vi "Scale Channel (Array).vi"(9 "Data":dbl[](array[numeric]), 10 "Scaling Params":dbl[](array[numeric]), 11 "Scaling Type":T1) -> (1 "Scaled Data":dbl[](array[numeric]))   [LabVIEW 2020, in "VolatusData.lvlib" / "Scaling.lvclass"]
uses:
  Scaling.lvclass
  Scaling.lvclass/Scaling.ctl
  VolatusConfig/Scale Type.ctl
  VolatusConfig/VolatusConfig.lvlib
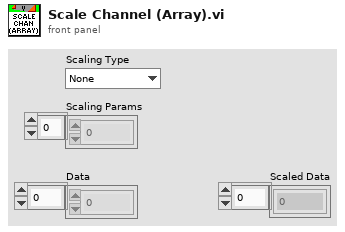
[diagram p1: front panel]
types:
  T1 = typedef "VolatusConfig.lvlib/Scale Type.ctl" = enum16{"None", "Sensor", "Polynomial", "Threshold", "Invert Bool"}
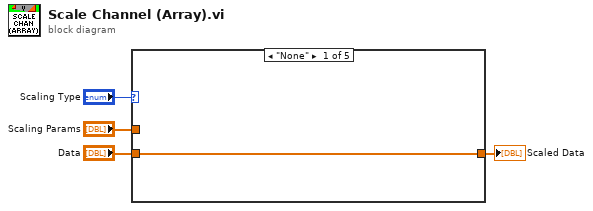
[diagram p0: block diagram]
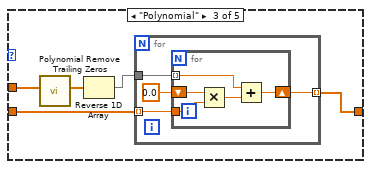
[diagram p3: hidden frame]
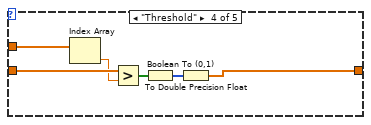
[diagram p4: hidden frame]
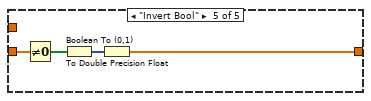
[diagram p5: hidden frame]
diagram:
  n1 = case shown="\"None\"" "Scaling Type" {
    tunnel: "Scaling Params" -> [_ _ w10 w26 _]
    tunnel: "Data" -> [w5 w6 w9 w25 w30]
    tunnel: [w5 w6 w7 w21 w27] -> w1
    frame "None" {
    }
    frame "Sensor" {
      # "#ERROR?\nSensor should be converted to another type."
    }
    frame "Polynomial" {
      n2 = call "Polynomial Remove Trailing Zeros.vi"("Coefficients"=w10) -> ("Used Coefficients"=w11:dbl[])  [unwired: 10 in]
      n3 = Reverse 1D Array(array=w11) -> (reversed array=w8:dbl[])
      n4 = for {
        tunnel: w9 -> [w14] mode=indexing
        tunnel: w8 -> [w13]
        tunnel: [w12] -> w7 mode=indexing
        n5 = for {
          tunnel: w13 -> [w17] mode=indexing
          tunnel: w14 -> [w19]
          shift-right: [w16] -> w12
          shift-left: 0.0 -> [w20]
          n6 = Multiply(x=w20, y=w19) -> (x*y=w18:dbl)
          n7 = Add(x=w17, y=w18) -> (x+y=w16:dbl)
        }
      }
    }
    frame "Threshold" {
      n8 = Index Array(array=w26) -> (element=w24:dbl)  [unwired: 1 in]
      n9 = Greater?(x=w25, y=w24) -> (0:w23:bool[])
      n10 = Boolean To (0,1)(Boolean=w23) -> (0, 1=w22:i16[])
      n11 = To Double Precision Float(number=w22) -> (double precision float=w21:dbl[])
    }
    frame "Invert Bool" {
      n12 = Not Equal To 0?(x=w30) -> (x != 0?=w29:bool[])
      n13 = Boolean To (0,1)(Boolean=w29) -> (0, 1=w28:i16[])
      n14 = To Double Precision Float(number=w28) -> (double precision float=w27:dbl[])
    }
  }
  "Scaled Data" <- w1
